vi "PID Convert.vi"(11 "PID gains in":T1) -> (3 "PID gains out":T2)   [LabVIEW 2013]
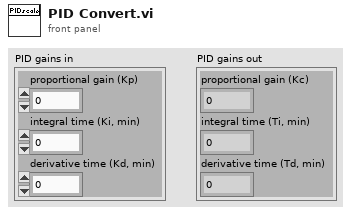
[diagram p1: front panel]
types:
  T1 = cluster{"proportional gain (Kp)":dbl, "integral time (Ki, min)":dbl, "derivative time (Kd, min)":dbl}
  T2 = cluster{"proportional gain (Kc)":dbl, "integral time (Ti, min)":dbl, "derivative time (Td, min)":dbl}
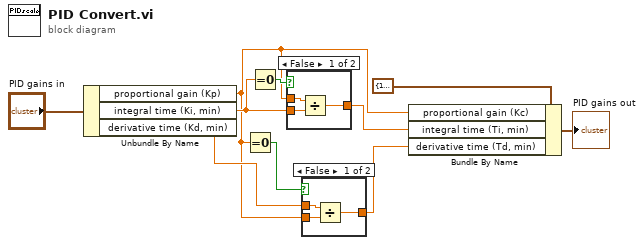
[diagram p0: block diagram]
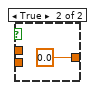
[diagram p2: hidden frame]
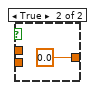
[diagram p3: hidden frame]
diagram:
  n1 = Unbundle By Name("PID gains in") -> ("proportional gain (Kp)"=w3:dbl, "integral time (Ki, min)"=w6:dbl, "derivative time (Kd, min)"=w4:dbl)
  n2 = Equal To 0?(x=w3) -> (x = 0?=w2:bool)
  n3 = Equal To 0?(x=w6) -> (x = 0?=w5:bool)
  n4 = case shown="False" w5 {
    tunnel: [w13 0.0] -> w9
    tunnel: w3 -> [w12 _]
    tunnel: w6 -> [w11 _]
    frame False {
      n5 = Divide(x=w12, y=w11) -> (x/y=w13:dbl)
    }
    frame True {
    }
  }
  n6 = case shown="False" w2 {
    tunnel: [w17 0.0] -> w1
    tunnel: w4 -> [w16 _]
    tunnel: w3 -> [w15 _]
    frame False {
      n7 = Divide(x=w16, y=w15) -> (x/y=w17:dbl)
    }
    frame True {
    }
  }
  n8 = Bundle By Name(cluster=T2 {"proportional gain (Kc)"=1.0, "integral time (Ti, min)"=0.01, "derivative time (Td, min)"=0.0} ("PID gains"), "proportional gain (Kc)"=w3, "integral time (Ti, min)"=w9, "derivative time (Td, min)"=w1) -> (→"PID gains out":T2)
